vi "转速测量2.vi"(1 "采样频率":dbl, 2 "阈值":dbl, 3 "转速数组":dbl[](array[numeric])) -> (0 "转速":dbl)   [LabVIEW 2014]
panel:
  in  "周期时刻数组":dbl[](array[numeric])
  in  "?":dbl
  # "周期计数"
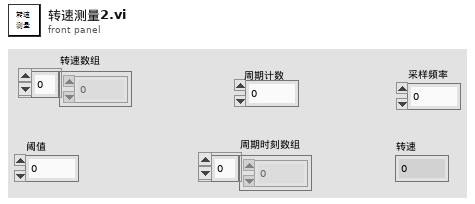
[diagram p1: front panel]
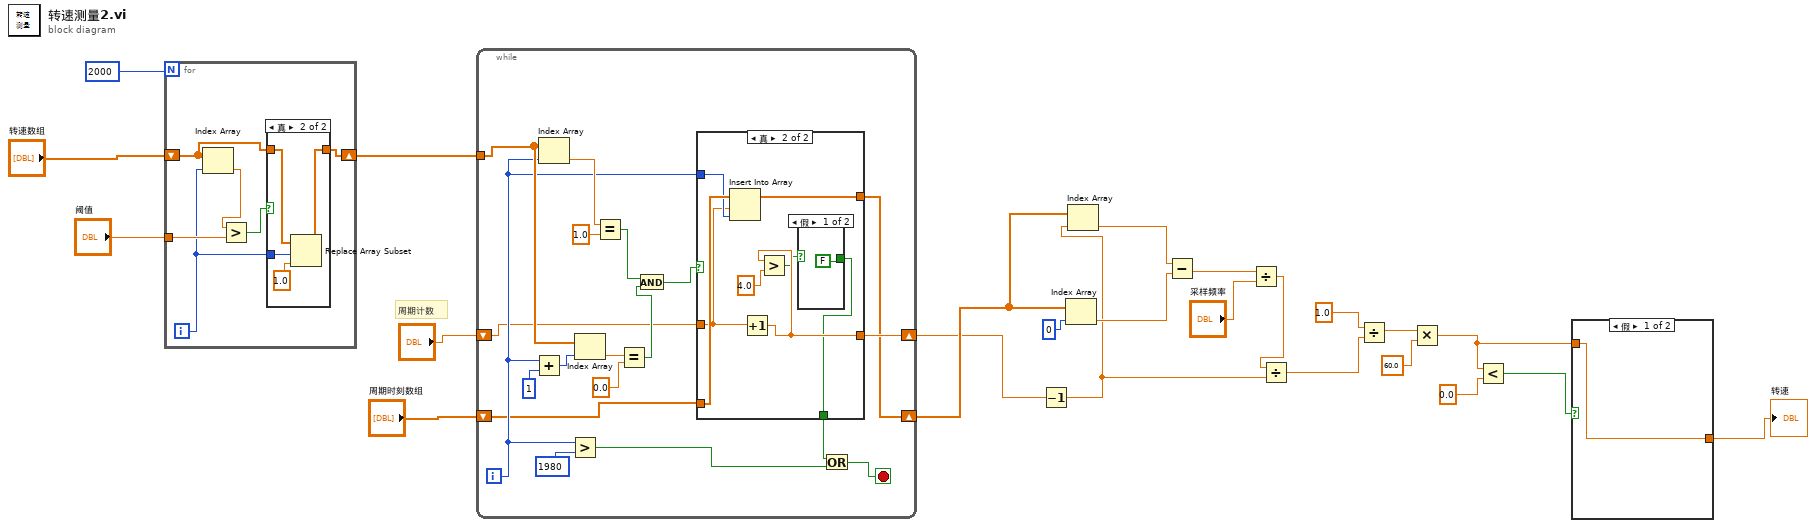
[diagram p0: block diagram]
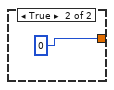
[diagram p2: hidden frame]
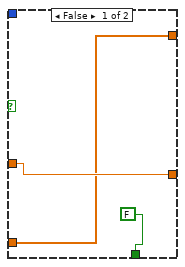
[diagram p3: hidden frame]
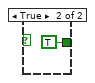
[diagram p4: hidden frame]
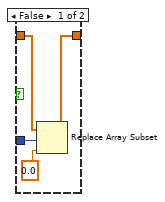
[diagram p5: hidden frame]
diagram:
  # "周期计数"
  n1 = for {
    N: 2000 -> [_]
    shift-right: [w24] -> w20
    shift-left: "转速数组" -> [w26]
    tunnel: "阈值" -> [w29]
    i -> [w25]
    n2 = Index Array(array=w26, index=w25) -> (element=w28:dbl)
    n3 = Greater?(x=w28, y=w29) -> (0:w27:bool)
    n4 = case shown="真" w27 {
      tunnel: w26 -> [w31 w37]
      tunnel: w25 -> [w33 w36]
      tunnel: [w30 w34] -> w24
      frame False {
        n5 = Replace Array Subset(array=w31, new element=0.0, index=w33) -> (w30:dbl[])
      }
      frame True {
        n6 = Replace Array Subset(array=w37, new element=1.0, index=w36) -> (w34:dbl[])
      }
    }
  }
  n7 = while {
    tunnel: w20 -> [w52]
    shift-right: [w41] -> w15
    shift-left: "?" -> [w42]
    shift-right: [w40] -> w17
    shift-left: "周期时刻数组" -> [w43]
    i -> [w46]
    stop <- w39 stop-if-true
    n8 = Add(x=w46, y=1) -> (x+y=w54:i32)
    n9 = Index Array(array=w52, index=w46) -> (element=w55:dbl)
    n10 = Greater?(x=w46, y=1980) -> (0:w44:bool)
    n11 = Index Array(array=w52, index=w54) -> (element=w51:dbl)
    n12 = Equal?(x=w55, y=1.0) -> (x = y?=w48:bool)
    n13 = Equal?(x=w51, y=0.0) -> (x = y?=w47:bool)
    n14 = And(x=w48, y=w47) -> (x .and. y?=w49:bool)
    n15 = case shown="真" w49 {
      tunnel: w46 -> [_ w61]
      tunnel: w43 -> [w58 w67]
      tunnel: w42 -> [w59 w60]
      tunnel: [w59 w64] -> w41
      tunnel: [w58 w66] -> w40
      tunnel: [FALSE w62] -> w38
      frame False {
      }
      frame True {
        n16 = Insert Into Array(array=w67, index=w60, new element=w61) -> (w66:dbl[])
        n17 = Increment(x=w60) -> (x+1=w64:dbl)
        n18 = Greater?(x=w64, y=4.0) -> (0:w63:bool)
        n19 = case shown="假" w63 {
          tunnel: [FALSE TRUE] -> w62
          frame False {
          }
          frame True {
          }
        }
      }
    }
    n20 = Or(x=w38, y=w44) -> (x .or. y?=w39:bool)
  }
  n21 = Decrement(x=w15) -> (x-1=w9:dbl)
  n22 = Index Array(array=w17, index=0) -> (element=w13:dbl)
  n23 = Index Array(array=w17, index=w9) -> (element=w14:dbl)
  n24 = Subtract(x=w14, y=w13) -> (x-y=w12:dbl)
  n25 = Divide(x=w12, y="采样频率") -> (x/y=w10:dbl)
  n26 = Divide(x=w10, y=w9) -> (x/y=w8:dbl)
  n27 = Divide(x=1.0, y=w8) -> (x/y=w6:dbl)
  n28 = Multiply(x=w6, y=60.0) -> (x*y=w2:dbl)
  n29 = Less?(x=w2, y=0.0) -> (x < y?=w3:bool)
  n30 = case shown="假" w3 {
    tunnel: w2 -> [w70 _]
    tunnel: [w70 0] -> w1
    frame False {
    }
    frame True {
    }
  }
  "转速" <- w1
